vi "Handle Command.vi"(8 "error in (no error)":errorcluster, 9 "Data":variant, 10 "Command":string, 11 "instrument.PPMS in":refnum<class "instrument.PPMS.lvclass">) -> (0 "error out":errorcluster, 1 "Processed Data":variant, 2 "Command":string, 3 "instrument.PPMS out":refnum<class "instrument.PPMS.lvclass">)   [LabVIEW 2016, in "instrument.PPMS.lvclass"]
uses:
  instrument.PPMS.lvclass
  Typedefs/PPMS.Magnet Field--cluster.ctl
  Typedefs/PPMS.Temperature--cluster.ctl
  <userlib>/LevyLab/Levylab Instruments/Instrument Types/Cryostat/Typedefs/Magnet Mode--Enum.ctl
  <userlib>/LevyLab/Levylab Instruments/Instrument Types/Cryostat/Instrument.Cryostat.lvclass
  Typedefs/PPMS.Magnet Status--cluster.ctl
  Typedefs/PPMS.Temperature Status--cluster.ctl
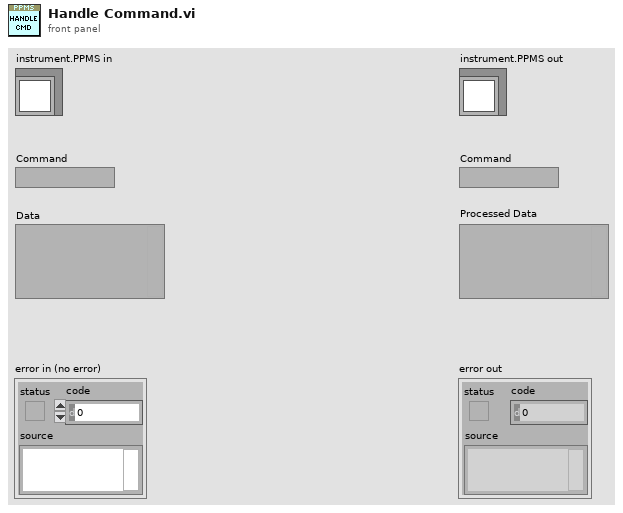
[diagram p1: front panel]
types:
  T1 = typedef "instrument.PPMS.lvclass/PPMS.Temperature--cluster.ctl" = cluster{"Temperature (K)":dbl, "Rate (K/min)":dbl}
  T2 = typedef "instrument.PPMS.lvclass/PPMS.Magnet Field--cluster.ctl" = cluster{"Target Field (Oe)":dbl, "Target Rate (Oe/s)":dbl, "Mode":T3}
  T3 = typedef "Instrument.Cryostat.lvclass/Magnet Mode--Enum.ctl" = enum16{"Persistent", "Driven"}
  T4 = typedef "instrument.PPMS.lvclass/PPMS.Magnet Status--cluster.ctl" = cluster{"Field (Oe)":dbl, "Magnet Status":string}
  T5 = typedef "instrument.PPMS.lvclass/PPMS.Temperature Status--cluster.ctl" = cluster{"Temperature (K)":dbl, "Temperature Status":string}
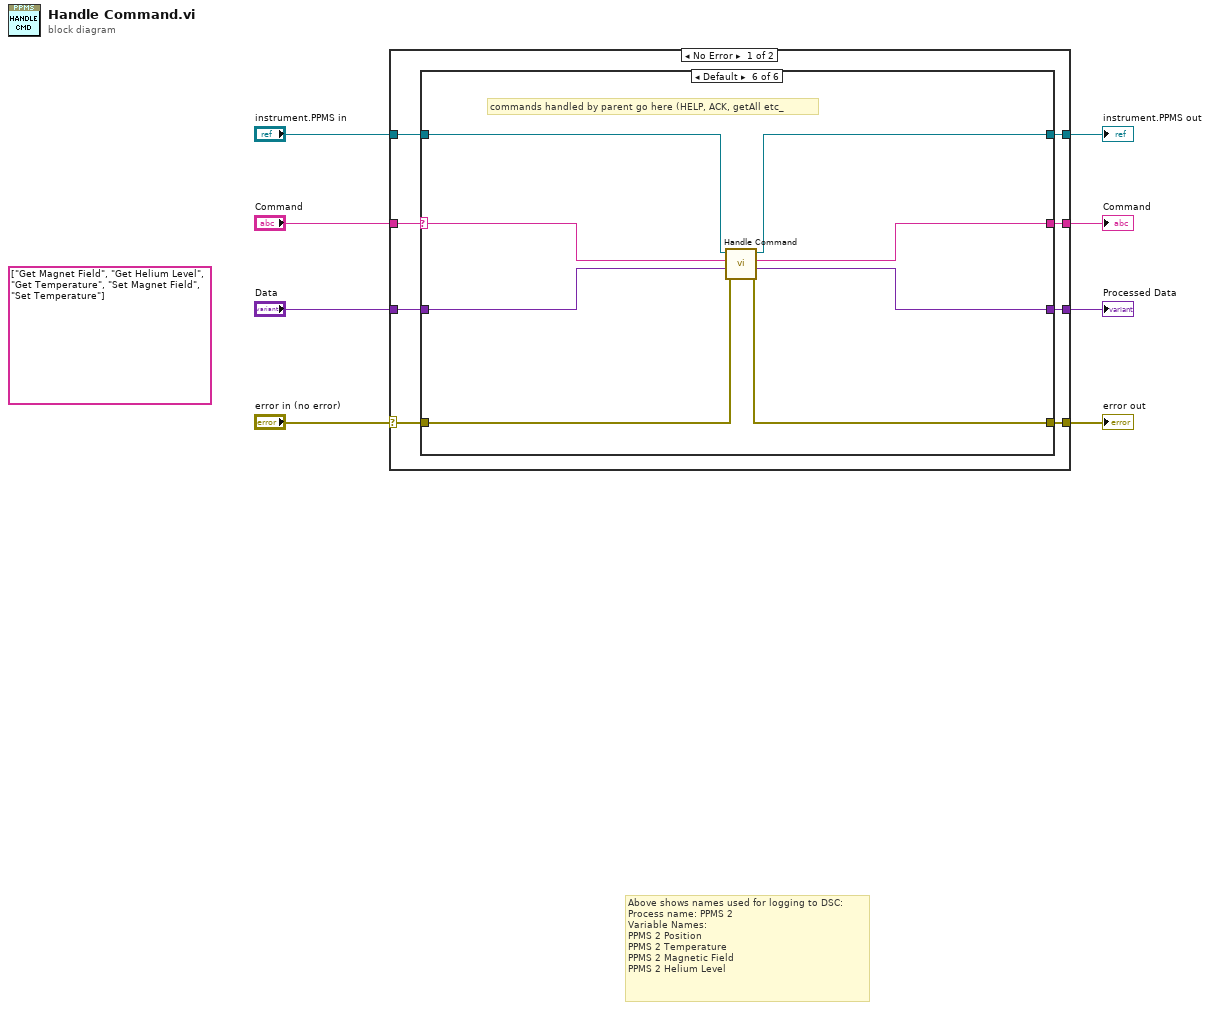
[diagram p0: block diagram]
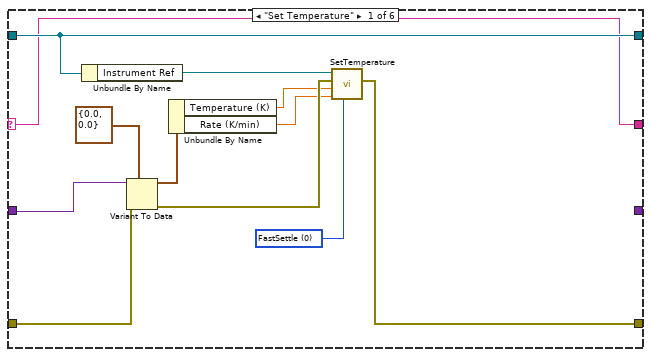
[diagram p2: hidden frame]
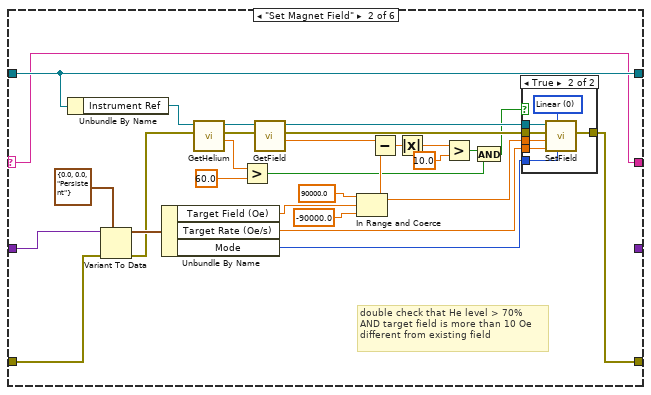
[diagram p3: hidden frame]
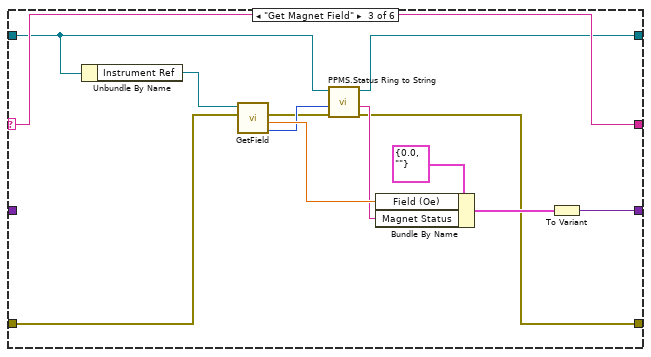
[diagram p5: hidden frame]
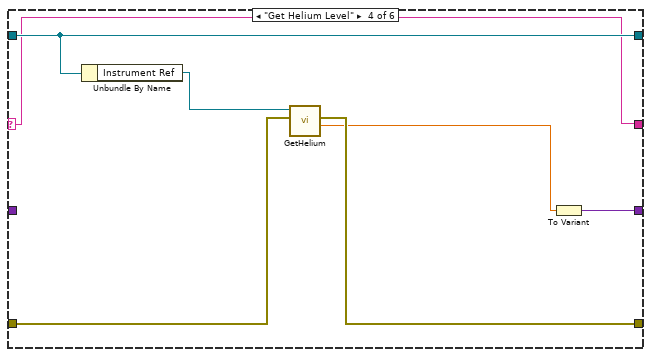
[diagram p6: hidden frame]
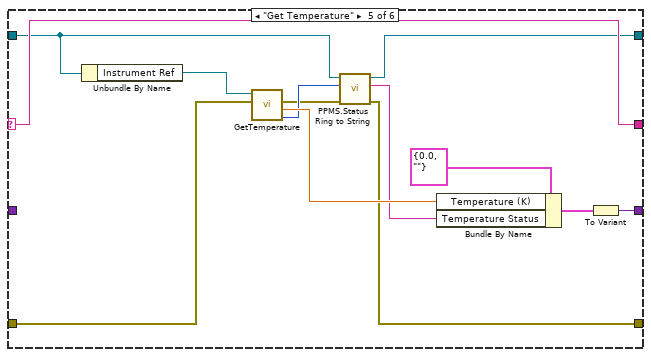
[diagram p7: hidden frame]
diagram:
  (unwired) string[] ["Get Magnet Field", "Get Helium Level", "Get Temperature", "Set Magnet Field", "Set Temperature"] ("Commands")
  # "Above shows names used for logging to DSC:\nProcess name: PPMS 2\nVariable Names:\nPPMS 2 Position\nPPMS 2 Temperature\nPPMS 2 Magnetic Field\nPPMS 2 Helium Level"
  n1 = case shown="No Error" "error in (no error)" {
    selector: "error in (no error)" -> [w11 w106]
    tunnel: [w10 w106] -> w6
    tunnel: [w16 _] -> w4
    tunnel: [w15 _] -> w5
    tunnel: [w14 w107] -> w7
    tunnel: "Data" -> [w13 _]
    tunnel: "Command" -> [w9 _]
    tunnel: "instrument.PPMS in" -> [w12 w107]
    frame No Error {
      n2 = case shown="Default" w9 {
        selector: w9 -> [w17 w30 w71 w78 w91 w98]
        tunnel: [_ _ w72 w80 w95 w105] -> w16
        tunnel: [w17 w30 w71 w78 w91 w104] -> w15
        tunnel: [w28 w56 w65 w84 w88 w103] -> w14
        tunnel: w13 -> [w23 w54 _ _ _ w102]
        tunnel: w12 -> [w28 w56 w66 w84 w89 w101]
        tunnel: w11 -> [w25 w53 w76 w83 w96 w100]
        tunnel: [w26 w51 w67 w82 w86 w99] -> w10
        frame "Set Temperature" {
          w18 = 0 items=["FastSettle", "NoOvershoot"] ("Approach")
          n3 = Unbundle By Name(w28) -> ("Instrument Ref"=w27:refnum<k24>)
          n4 = Variant To Data(error in=w25, type=T1 {"Temperature (K)"=0.0, "Rate (K/min)"=0.0} ("Temperature"), Variant=w23) -> (data=w22:T1, error out=w21:errorcluster)
          n5 = Unbundle By Name(w22) -> ("Temperature (K)"=w20:dbl, "Rate (K/min)"=w19:dbl)
          n6 = call "SetTemperature.vi"("Approach"=w18, "Rate"=w19, "Temperature"=w20, "error in (no error)"=w21, "Instrument Ref In"=w27) -> ("error out"=w26:errorcluster)  [unwired: 2 in, 2 out]
        }
        frame "Set Magnet Field" {
          # "double check that He level > 70%\nAND target field is more than 10 Oe\ndifferent from existing field"
          n7 = Unbundle By Name(w56) -> ("Instrument Ref"=w29:refnum<k24>)
          n8 = Variant To Data(error in=w53, type=T2 {"Target Field (Oe)"=0.0, "Target Rate (Oe/s)"=0.0, "Mode"=enum."Persistent"} ("Magnet Field"), Variant=w54) -> (data=w52:T2, error out=w50:errorcluster)
          n9 = Unbundle By Name(w52) -> ("Target Field (Oe)"=w40:dbl, "Target Rate (Oe/s)"=w43:dbl, "Mode"=w32:T3)
          n10 = call "GetHelium.vi"("error in (no error)"=w50, "Instrument Refnum in"=w29) -> ("Helium Level (%)"=w44:dbl, "error out"=w49:errorcluster, "Instrument Ref Out"=w47:refnum<k24>)  [unwired: 3 in]
          n11 = Greater?(x=w44, y=60.0) -> (0:w33:bool)
          n12 = call "GetField.vi"("error in (no error)"=w49, "Instrument Ref In"=w47) -> ("Field"=w36:dbl, "error out"=w48:errorcluster, "Instrument Ref Out"=w46:refnum<k24>)  [unwired: 3 in, 2 out]
          n13 = In Range and Coerce(upper limit=90000.0, x=w40, lower limit=-90000.0) -> (coerced(x)=w37:dbl)  [unwired: 1 out]
          n14 = Subtract(x=w36, y=w37) -> (x-y=w35:dbl)
          n15 = Absolute Value(x=w35) -> (abs(x)=w39:dbl)
          n16 = Greater?(x=w39, y=10.0) -> (0:w34:bool)
          n17 = And(x=w34, y=w33) -> (x .and. y?=w31:bool)
          n18 = case shown="True" w31 {
            tunnel: [w57 w63] -> w51
            tunnel: w48 -> [w57 w62]
            tunnel: w46 -> [_ w61]
            tunnel: w43 -> [_ w60]
            tunnel: w37 -> [_ w59]
            tunnel: w32 -> [_ w58]
            frame False {
            }
            frame True {
              w64 = 0 items=["Linear", "NoOvershoot", "Oscillate"] ("Approach")
              n19 = call "SetField.vi"("Mode"=w58, "Approach"=w64, "Rate"=w60, "Field"=w59, "error in (no error)"=w62, "Instrument Ref In"=w61) -> ("error out"=w63:errorcluster)  [unwired: 1 in, 2 out]
            }
          }
        }
        frame "Get Magnet Field" {
          n20 = Unbundle By Name(w66) -> ("Instrument Ref"=w77:refnum<k24>)
          n21 = call "GetField.vi"("error in (no error)"=w76, "Instrument Ref In"=w77) -> ("Field\nStatus"=w70:i32, "Field"=w75:dbl, "error out"=w68:errorcluster)  [unwired: 3 in, 2 out]
          n22 = call "PPMS.Status Ring to String.vi"("error in (no error)"=w68, "Field Status"=w70, "instrument.PPMS in"=w66) -> ("error out"=w67:errorcluster, "Field Status String"=w69:string, "instrument.PPMS out"=w65:refnum<class "instrument.PPMS.lvclass">)  [unwired: 5 in, 1 out]
          n23 = Bundle By Name(cluster=T4 {"Field (Oe)"=0.0, "Magnet Status"=""}, "Field (Oe)"=w75, "Magnet Status"=w69) -> (w73:T4)
          n24 = To Variant(anything=w73) -> (Variant=w72:variant)
        }
        frame "Get Helium Level" {
          n25 = Unbundle By Name(w84) -> ("Instrument Ref"=w79:refnum<k24>)
          n26 = call "GetHelium.vi"("error in (no error)"=w83, "Instrument Refnum in"=w79) -> ("Helium Level (%)"=w81:dbl, "error out"=w82:errorcluster)  [unwired: 3 in, 1 out]
          n27 = To Variant(anything=w81) -> (Variant=w80:variant)
        }
        frame "Get Temperature" {
          n28 = Unbundle By Name(w89) -> ("Instrument Ref"=w97:refnum<k24>)
          n29 = call "GetTemperature.vi"("error in (no error)"=w96, "Instrument Ref In"=w97) -> ("Temperature\nStatus"=w90:i32, "Temperature"=w94:dbl, "error out"=w87:errorcluster)  [unwired: 3 in, 2 out]
          n30 = call "PPMS.Status Ring to String.vi"("error in (no error)"=w87, "Temperature Status"=w90, "instrument.PPMS in"=w89) -> ("error out"=w86:errorcluster, "Temperature Status String"=w85:string, "instrument.PPMS out"=w88:refnum<class "instrument.PPMS.lvclass">)  [unwired: 5 in, 1 out]
          n31 = Bundle By Name(cluster=T5 {"Temperature (K)"=0.0, "Temperature Status"=""}, "Temperature (K)"=w94, "Temperature Status"=w85) -> (w92:T5)
          n32 = To Variant(anything=w92) -> (Variant=w95:variant)
        }
        frame Default {
          # "commands handled by parent go here (HELP, ACK, getAll etc_"
          n33 = call-parent "Handle Command.vi"("error in (no error)"=w100, "Data"=w102, "Command"=w98, "Instrument in"=w101) -> ("error out"=w99:errorcluster, "Processed Data"=w105:variant, "Command"=w104:string, "Instrument out"=w103:refnum<class "instrument.PPMS.lvclass">)  [unwired: 4 in]
        }
      }
    }
    frame Error {
    }
  }
  "error out" <- w6
  "instrument.PPMS out" <- w7
  "Processed Data" <- w4
  "Command" <- w5
